vi "Append Front Panel Image to Report (path).vi"(0 "report in":refnum<class "NI_report.lvclass">, 1 "alignment (default)":T2, 2 "image format (jpeg)":enum32{"PNG", "JPEG", "GIF"}(ring)=enum."JPEG", 5 "VI":path, 9 "description":string, 11 "error in (no error)":errorcluster, 12 "visible area only?":bool, 13 "MS Office parameters":T1) -> (4 "report out":refnum<class "NI_report.lvclass">, 6 "VI path out":path, 8 "start out (Word)":i32, 10 "end out (Word)":i32, 15 "error out":errorcluster)   [LabVIEW 2020, in "NI_ReportGenerationCore.lvlib"]
doc: "Creates an image of the front panel of the VI you specify in <B>VI</B> and appends it to a report. Wire data to the <B>VI</B> input to determine the polymorphic instance to use or manually select the instance."
uses:
  <vilib>/Utility/NIReport.llb/NI_ReportGenerationCore.lvlib
  <vilib>/Utility/NIReport.llb/NI_report.lvclass
  <vilib>/Utility/NIReport.llb/HTML Report Image Alignment.ctl
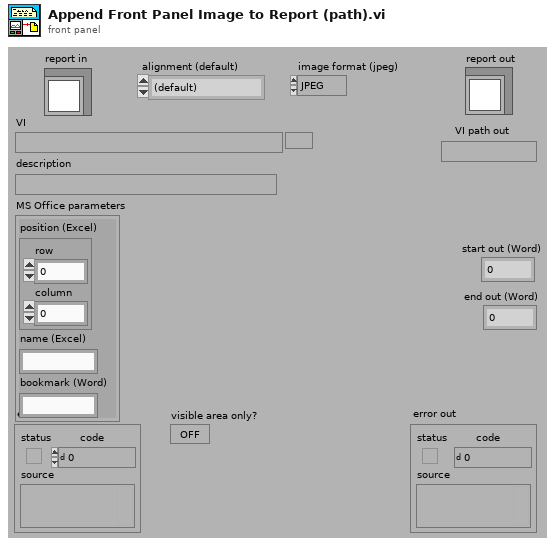
[diagram p1: front panel]
types:
  T1 = cluster{"position (Excel)":cluster{"row":i32, "column":i32}, "name (Excel)":string, "bookmark (Word)":string}
  T2 = typedef "NI_ReportGenerationCore.lvlib/HTML Report Image Alignment.ctl" = enum16{"(default)", "LEFT", "RIGHT", "TOP", "TEXTTOP", "MIDDLE", "ABSMIDDLE", "BASELINE", "BOTTOM", "ABSBOTTOM"}
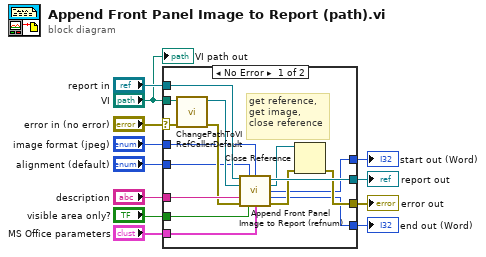
[diagram p0: block diagram]
diagram:
  n1 = case shown="No Error" "error in (no error)" {
    selector: "error in (no error)" -> [w22 w30]
    tunnel: [w15 w30] -> w11
    tunnel: "report in" -> [w26 w29]
    tunnel: "VI" -> [w28 _]
    tunnel: "description" -> [w25 _]
    tunnel: "visible area only?" -> [w23 _]
    tunnel: "alignment (default)" -> [w21 _]
    tunnel: [w20 w29] -> w5
    tunnel: "MS Office parameters" -> [w19 _]
    tunnel: "image format (jpeg)" -> [w18 _]
    tunnel: [w14 _] -> w2
    tunnel: [w13 _] -> w1
    frame No Error {
      # "get reference,\nget image,\nclose reference"
      n2 = call <vilib>:"ChangePathToVIRefCallerDefault.vi"("error in (no error)"=w22, "VI path"=w28) -> ("error out"=w24:errorcluster, "VI reference"=w27:refnum<vi>)  [unwired: 4 in]
      n3 = call <vilib>:"Append Front Panel Image to Report (refnum).vi"("report in"=w26, "alignment (default)"=w21, "image format (jpeg)"=w18, "VI"=w27, "description"=w25, "error in (no error)"=w24, "visible area only?"=w23, "MS Office parameters"=w19) -> ("report out"=w20:refnum<class "NI_report.lvclass">, "VI out"=w17:refnum<vi>, "start out (Word)"=w14:i32, "end out (Word)"=w13:i32, "error out"=w16:errorcluster)  [unwired: 3 in]
      n4 = Close Reference(reference=w17, error in (no error)=w16) -> (error out=w15:errorcluster)
    }
    frame Error {
    }
  }
  "error out" <- w11
  "report out" <- w5
  "start out (Word)" <- w2
  "end out (Word)" <- w1
  "VI path out" <- "VI"
